vi "Change FP Items Properties.vi"(6 "Select FP Item In":T1, 7 "Properties in":T2, 8 "error in (no error)":errorcluster, 10 "VI in":refnum<vi>, 11 "Boolean in":refnum<vi>) -> (0 "error out":errorcluster, 3 "VI out":refnum<vi>)   [LabVIEW 2020]
uses:
  TDefs/FP Items Properties.ctl
  TDefs/Selected FP Items.ctl
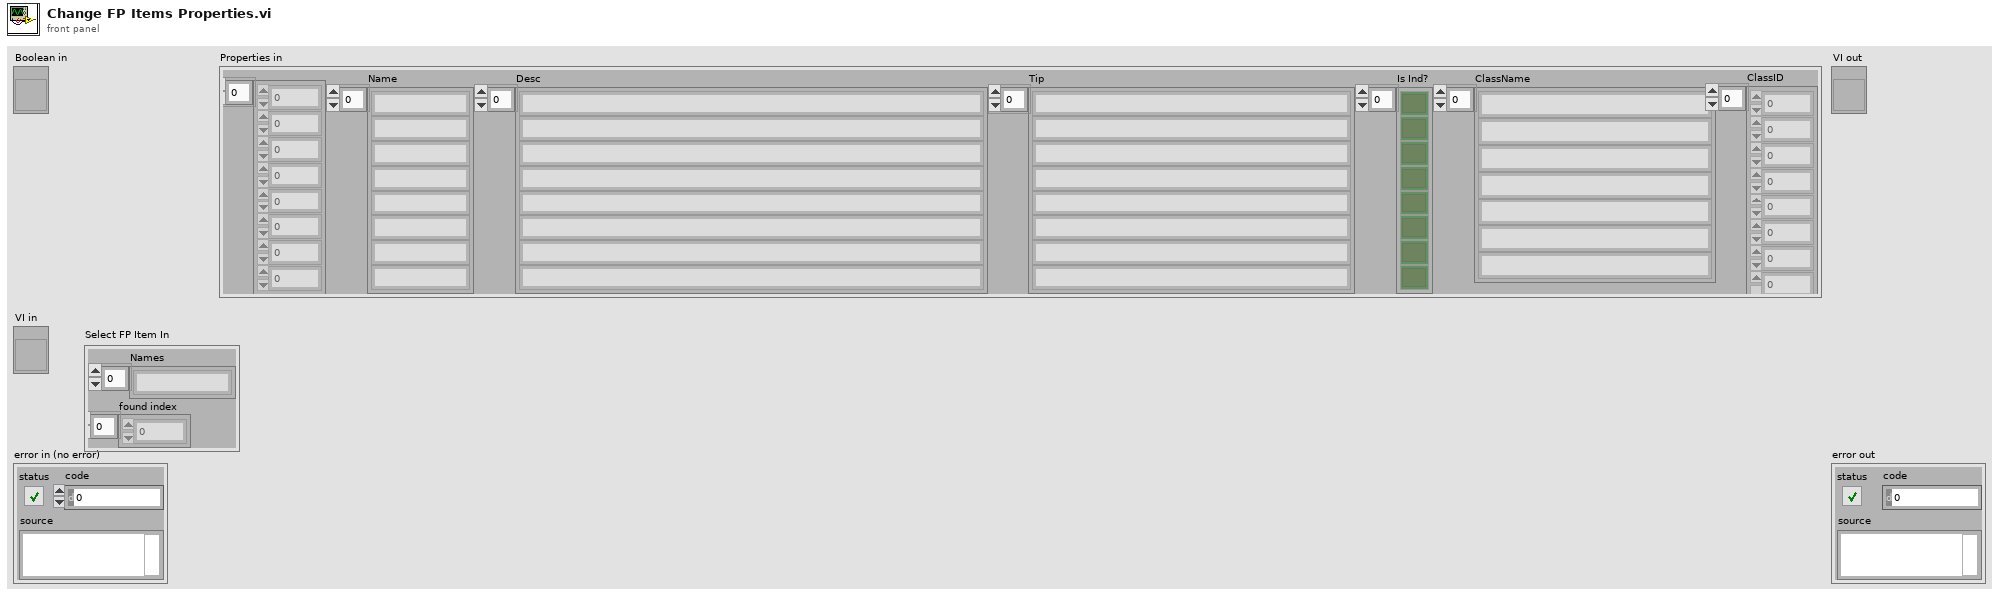
[diagram p1: front panel]
types:
  T1 = typedef "Selected FP Items.ctl" = cluster{"Names":string[], "found index":i32[]}
  T2 = typedef "FP Items Properties.ctl" = cluster{"index":i32[], "Name":string[], "Desc":string[], "Tip":string[], "Is Ind?":bool[], "ClassName":string[], "ClassID":u32[]}
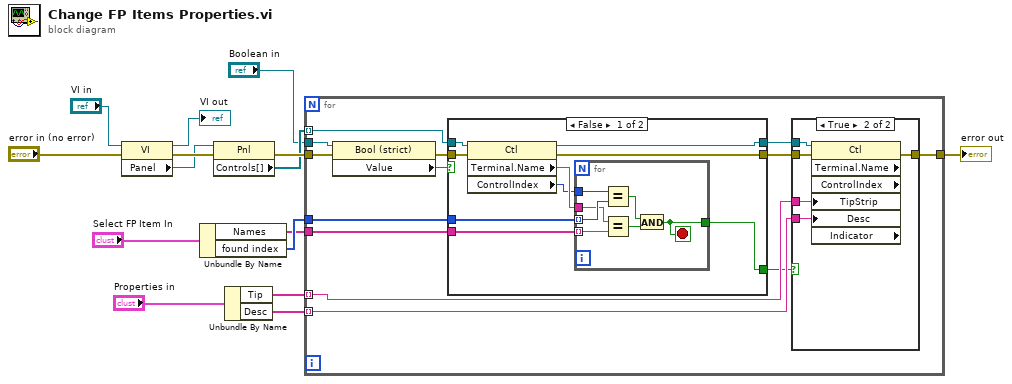
[diagram p0: block diagram]
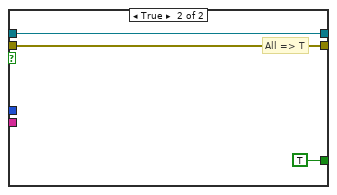
[diagram p2: hidden frame]
diagram:
  n1 = property class="VI"(reference="VI in", error in="error in (no error)") -> (reference out=→"VI out":refnum<vi>, error out=w8:errorcluster, "Panel"=w5:refnum<vi>)
  n2 = Unbundle By Name("Select FP Item In") -> ("Names"=w1:string[], "found index"=w2:i32[])
  n3 = property class="Pnl"(reference=w5, error in=w8) -> (error out=w7:errorcluster, "Controls[]"=w6:refnum<vi>[])  [unwired: 1 out]
  n4 = Unbundle By Name("Properties in") -> ("Tip"=w14:string[], "Desc"=w15:string[])
  n5 = for {
    tunnel: w6 -> [w20] mode=indexing
    tunnel: w14 -> [w28] mode=indexing
    tunnel: w15 -> [w27] mode=indexing
    tunnel: w7 -> [w19]
    tunnel: [w26] -> w12
    tunnel: w2 -> [w25]
    tunnel: w1 -> [w24]
    tunnel: "Boolean in" -> [w16]
    n6 = property on="Property Node" class="Bool (strict)"(reference=w16, error in=w19) -> (error out=w18:errorcluster, "Value"=w17:bool)  [unwired: 1 out]
    n7 = case shown="False" w17 {
      tunnel: w25 -> [w37 _]
      tunnel: w24 -> [w36 _]
      tunnel: [w33 TRUE] -> w23
      tunnel: [w32 w46] -> w22
      tunnel: [w31 w47] -> w21
      tunnel: w20 -> [w30 w47]
      tunnel: w18 -> [w29 w46]
      frame False {
        n8 = property class="Ctl"(reference=w30, error in=w29) -> (reference out=w31:refnum<vi>, error out=w32:errorcluster, "Terminal.Name"=w35:string, "ControlIndex"=w34:i32)
        n9 = for {
          tunnel: w37 -> [w43] mode=indexing
          tunnel: w36 -> [w41] mode=indexing
          tunnel: w35 -> [w42]
          tunnel: w34 -> [w44]
          tunnel: [w38] -> w33
          stop <- w38 stop-if-true
          n10 = Equal?(x=w44, y=w43) -> (x = y?=w40:bool)
          n11 = Equal?(x=w42, y=w41) -> (x = y?=w39:bool)
          n12 = And(x=w40, y=w39) -> (x .and. y?=w38:bool)
        }
      }
      frame True {
        # "All => T"
      }
    }
    n13 = case shown="True" w23 {
      tunnel: w21 -> [_ w53]
      tunnel: w28 -> [_ w52]
      tunnel: w27 -> [_ w51]
      tunnel: w22 -> [w48 w50]
      tunnel: [w48 w49] -> w26
      frame False {
      }
      frame True {
        n14 = property class="Ctl" props=["Terminal", "Name", "ControlIndex", "TipStrip", "Desc", "Indicator"](reference=w53, error in=w50, "TipStrip"=w52, "Desc"=w51) -> (error out=w49:errorcluster)  [unwired: 4 out]
      }
    }
  }
  "error out" <- w12
